vi "Teleop.vi"(10 "Match Info":T1={"Autonomous Elapsed Seconds"=0.0, "TeleOp Elapsed Seconds"=0.0, "Disabled Elapsed Seconds"=0.0, "Visited Autonomous"=FALSE, "Visited TeleOp"=FALSE, "Visited Disabled"=FALSE, "Autonomous Settings"={"Autonomous Style"=enum."Independent", "VI Refnum"=refnum}}, 11 "Call Context":T2) -> ()   [LabVIEW 2011]
doc: "This VI is called for each TeleOp packet received from the DS where the robot is not disabled. It is often used to read from the joysticks and update I/O or to update setpoints for timed control loops. It should complete and return within 20 milliseconds or it may miss DS packets."
uses:
  <vilib>/Rock Robotics/WPI/DriverStation/WPI_DriverStationDerivedRobotMode.ctl
  <vilib>/Rock Robotics/WPI/DriverStation/WPI_DriverStationMatch Info.ctl
  <vilib>/Rock Robotics/WPI/Relay/WPI_RelayValue.ctl
  <vilib>/Rock Robotics/WPI/DriverStation/DriverStationLCD/WPI_DriverStationLCDLCDLine.ctl
  Robot Global Data.vi
panel:
  in  "LDrive0":dbl
  in  "Rdrive0":dbl=0.9
  in  "Rdrive2":dbl=0.6
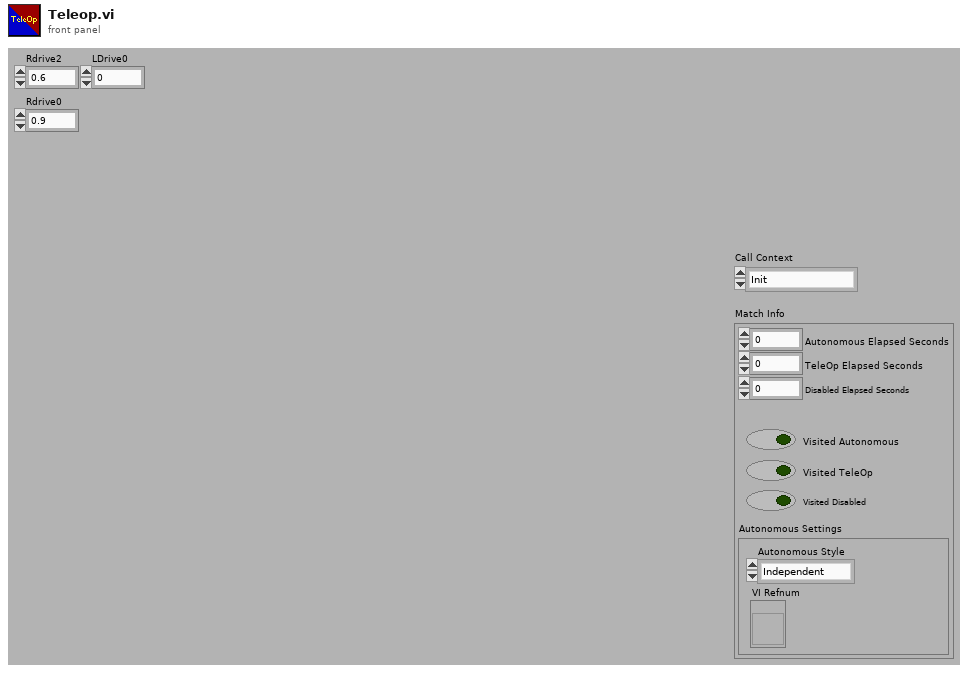
[diagram p1: front panel]
types:
  T1 = typedef "WPI_DriverStationMatch Info.ctl" = cluster{"Autonomous Elapsed Seconds":dbl, "TeleOp Elapsed Seconds":dbl, "Disabled Elapsed Seconds":dbl, "Visited Autonomous":bool, "Visited TeleOp":bool, "Visited Disabled":bool, "Autonomous Settings":cluster{"Autonomous Style":enum16{"Iterative", "Independent"}, "VI Refnum":refnum<vi>}}
  T2 = typedef "WPI_DriverStationDerivedRobotMode.ctl" = enum16{"Init", "Execute", "Stop"}
  T3 = typedef "WPI_RelayValue.ctl" = enum16{"Off", "On", "Forward", "Reverse"}
  T4 = typedef "WPI_JoystickDevRef.ctl" = cluster{"Device":T5}
  T5 = typedef "WPI_JoystickDeviceEnum.ctl" = enum16{"USB 1", "USB 2", "USB 3", "USB 4", "Kinect 1", "Kinect 2"}
  T6 = typedef "WPI_JoystickButtonState.ctl" = cluster{"Button 1":bool, "Button 2":bool, "Button 3":bool, "Button 4":bool, "Button 5":bool, "Button 6":bool, "Button 7":bool, "Button 8":bool, "Button 9":bool, "Button 10":bool, "Button 11":bool, "Button 12":bool}
  T7 = cluster{"axis 1 (x)":dbl, "axis 2 (y)":dbl, "axis 3 (throttle)":dbl, "axis 4":dbl, "axis 5":dbl, "axis 6":dbl}
  T8 = typedef "WPI_MotorControlDeviceRef.ctl" = cluster{"DeviceStatus":errorcluster, "Type":enum16{"PWM", "CAN"}, "PWM":cluster{"Digital Module":T9, "PWM Channel":T10, "DeadBand":T11}, "CAN":cluster{"Device Number":u8, "Control Mode":T12, "Semaphore":T13, "Max Vout":dbl}, "Invert":bool, "TransformRef":T14, "InvTransformRef":T14}
  T9 = typedef "FPGA_TypedefDigitalModule.ctl" = enum16{"Digital Module 1", "Digital Module 2"}
  T10 = typedef "FPGA_DIOPWMChannel.ctl" = enum8{"PWM 1", "PWM 2", "PWM 3", "PWM 4", "PWM 5", "PWM 6", "PWM 7", "PWM 8", "PWM 9", "PWM 10", "Invalid"}
  T11 = typedef "WPI_PWMDeadband.ctl" = cluster{"Name":string, "maxPositivePwm":i32, "minPositivePwm":i32, "centerPwm":i32, "maxNegativePwm":i32, "minNegativePwm":i32, "angularRange":u16}
  T12 = typedef "WPI_CANJaguar_ControlMode.ctl" = enum8{"Percent VBus", "Current", "Speed", "Position", "Voltage"}
  T13 = typedef "Semaphore RefNum" = refnum<k1>
  T14 = typedef "WPI_PWMTransform_ConPane.ctl" = refnum<vi>
  T15 = cluster{"Driver Station Digital Input (1-8)[0]":bool, "Driver Station Digital Input (1-8)[1]":bool, "Driver Station Digital Input (1-8)[2]":bool, "Driver Station Digital Input (1-8)[3]":bool, "Driver Station Digital Input (1-8)[4]":bool, "Driver Station Digital Input (1-8)[5]":bool, "Driver Station Digital Input (1-8)[6]":bool, "Driver Station Digital Input (1-8)[7]":bool, "Driver Station Digital Input (1-8)[8]":bool}
  T16 = typedef "WPI_RelayDevRef.ctl" = cluster{"DevStatus":errorcluster, "Relay Channel":T17, "Digital Module":T9, "Relay Direction":T18}
  T17 = typedef "FPGA_DIORelayChannel.ctl" = enum8{"Relay 1", "Relay 2", "Relay 3", "Relay 4", "Relay 5", "Relay 6", "Relay 7", "Relay 8", "Invalid"}
  T18 = typedef "WPI_RelayDirection.ctl" = enum16{"Both directions", "Forward only", "Reverse only"}
  T19 = typedef "WPI_DigitalInputDevRef.ctl" = cluster{"DevStatus":errorcluster, "DIO Channel":T20, "Digital Module":T9}
  T20 = typedef "FPGA_DIOChannel.ctl" = enum8{"DIO 1", "DIO 2", "DIO 3", "DIO 4", "DIO 5", "DIO 6", "DIO 7", "DIO 8", "DIO 9", "DIO 10", "DIO 11", "DIO 12", "DIO 13", "DIO 14", "Invalid"}
  T21 = typedef "WPI_EncoderDevRef.ctl" = cluster{"DevStatus":errorcluster, "EncoderIndex":T22, "CounterIndex":T23, "DistancePerCount":dbl, "Decoding Type":T24}
  T22 = typedef "FPGA_EncoderIdx.ctl" = enum8{"Enc 0", "Enc 1", "Enc 2", "Enc 3", "Invalid"}
  T23 = typedef "FPGA_CounterCtrSystemIndex.ctl" = enum8{"Ctr 0", "Ctr 1", "Ctr 2", "Ctr 3", "Ctr 4", "Ctr 5", "Ctr 6", "Ctr 7", "Invalid"}
  T24 = typedef "WPI_EncoderType.ctl" = enum16{"1x", "2x", "4x"}
  T25 = typedef "WPI_DriverStationLCDLCDLine.ctl" = enum16{"Main - Line 1", "User - Line 2", "User - Line 3", "User - Line 4", "User - Line 5", "User - Line 6"}
  T26 = typedef "WPI_ServoDeviceRef.ctl" = cluster{"DeviceStatus":errorcluster, "Digital Module":T9, "PWM Channel":T10, "DeadBand":T11}
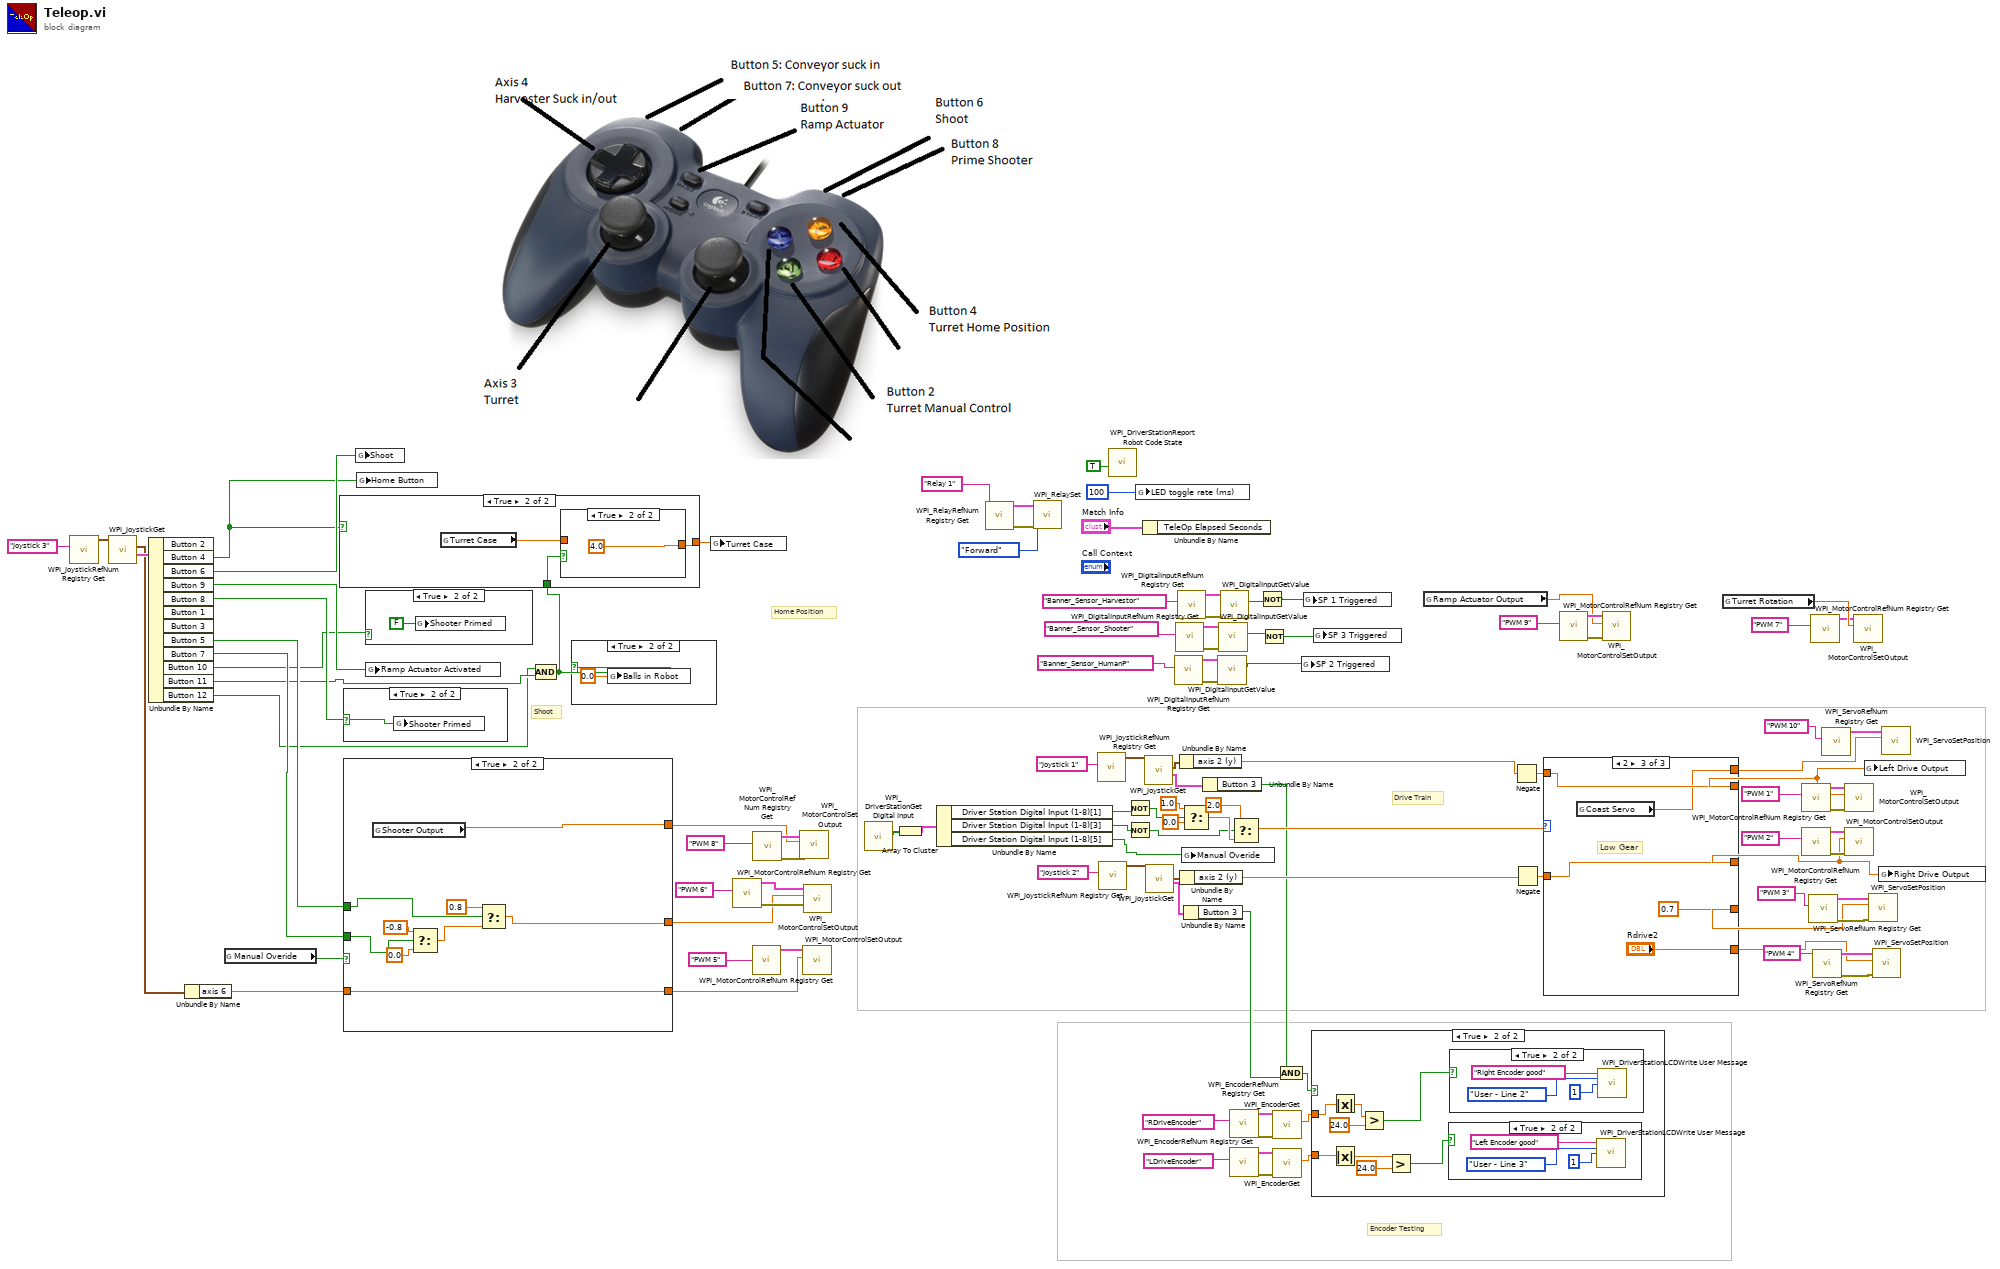
[diagram p0: block diagram]
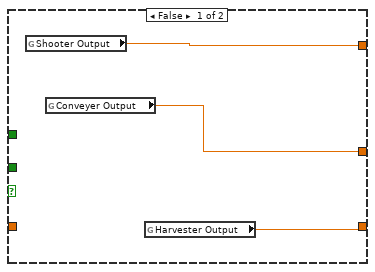
[diagram p7: hidden frame]
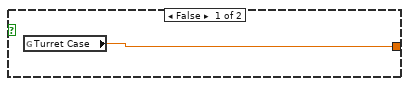
[diagram p9: hidden frame]
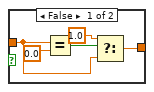
[diagram p10: hidden frame]
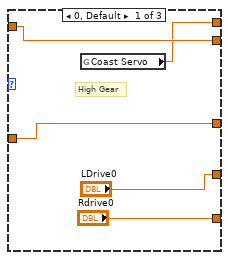
[diagram p11: hidden frame]
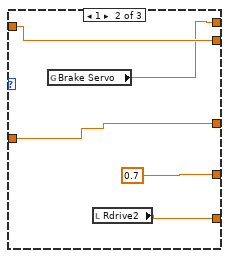
[diagram p12: hidden frame]
diagram:
  # "Encoder Testing"
  # "Shoot"
  # "Home Position"
  # "Drive Train"
  n1 = call <vilib>:"WPI_JoystickRefNum Registry Get.vi"("refnum name"="Joystick 3") -> ("JoystickDevRef"=w63:T4)  [unwired: 9 in, 1 out]
  n2 = call <vilib>:"WPI_JoystickGet.vi"("JoystickDevRef"=w63) -> ("Buttons"=w64:T6, "Axes"=w37:T7)  [unwired: 4 in, 1 out]
  n3 = Unbundle By Name(w64) -> ("Button 4"=w26:bool, "Button 6"=w62:bool, "Button 9"=w66:bool, "Button 8"=w38:bool, "Button 5"=w34:bool, "Button 7"=w33:bool, "Button 10"=w25:bool, "Button 11"=w24:bool, "Button 12"=w23:bool)  [unwired: 3 out]
  n4 = Unbundle By Name(w37) -> ("axis 6"=w21:dbl)
  n5 = global read "Robot Global Data.vi" "Manual Overide"() -> (w28:bool)
  n6 = case shown="True" w38 {
    selector: w38 -> [_ w111]
    frame False {
    }
    frame True {
      n7 = global write "Robot Global Data.vi" "Shooter Primed"(w111) -> ()
    }
  }
  n8 = case shown="True" w28 {
    tunnel: [w114 w115] -> w35
    tunnel: w34 -> [_ w118]
    tunnel: w33 -> [_ w119]
    tunnel: [w113 w117] -> w29
    tunnel: [w112 w116] -> w22
    tunnel: w21 -> [_ w116]
    frame False {
      n9 = global read "Robot Global Data.vi" "Shooter Output"() -> (w114:dbl)
      n10 = global read "Robot Global Data.vi" "Conveyer Output"() -> (w113:dbl)
      n11 = global read "Robot Global Data.vi" "Harvester Output"() -> (w112:dbl)
    }
    frame True {
      n12 = global read "Robot Global Data.vi" "Shooter Output"() -> (w115:dbl)
      n13 = Select(t=-0.8, s=w119, f=0.0) -> (s? t:f=w123:dbl)
      n14 = Select(t=0.8, s=w118, f=w123) -> (s? t:f=w117:dbl)
    }
  }
  n15 = global write "Robot Global Data.vi" "Shoot"(w62) -> ()
  n16 = global write "Robot Global Data.vi" "Home Button"(w26) -> ()
  n17 = case shown="True" w25 {
    frame False {
    }
    frame True {
      n18 = global write "Robot Global Data.vi" "Shooter Primed"(FALSE ("Shooter Primed")) -> ()
    }
  }
  n19 = global write "Robot Global Data.vi" "Ramp Actuator Activated"(w66) -> ()
  n20 = Compound Arithmetic op=AND(w23, w24) -> (w20:bool)
  n21 = case shown="True" w26 {
    tunnel: [w125 w126] -> w19
    tunnel: w20 -> [_ w128]
    frame False {
      n22 = global read "Robot Global Data.vi" "Turret Case"() -> (w125:dbl)
    }
    frame True {
      n23 = global read "Robot Global Data.vi" "Turret Case"() -> (w127:dbl)
      n24 = case shown="True" w128 {
        tunnel: w127 -> [w130 _]
        tunnel: [w129 4.0 ("Turret Case")] -> w126
        frame False {
          n25 = Equal?(x=w130, y=0.0) -> (x = y?=w132:bool)
          n26 = Select(t=1.0, s=w132, f=w130) -> (s? t:f=w129:dbl)
        }
        frame True {
        }
      }
    }
  }
  n27 = case shown="True" w20 {
    frame False {
    }
    frame True {
      n28 = global write "Robot Global Data.vi" "Balls in Robot"(0.0 ("Balls in Robot")) -> ()
    }
  }
  n29 = global write "Robot Global Data.vi" "Turret Case"(w19) -> ()
  n30 = call <vilib>:"WPI_MotorControlRefNum Registry Get.vi"("refnum name"="PWM 6") -> ("error out"=w30:errorcluster, "MotorControlDevRef"=w31:T8)  [unwired: 9 in]
  n31 = call <vilib>:"WPI_MotorControlRefNum Registry Get.vi"("refnum name"="PWM 5") -> ("MotorControlDevRef"=w56:T8)  [unwired: 9 in, 1 out]
  n32 = call <vilib>:"WPI_MotorControlRefNum Registry Get.vi"("refnum name"="PWM 8") -> ("error out"=w40:errorcluster, "MotorControlDevRef"=w41:T8)  [unwired: 9 in]
  n33 = call <vilib>:"WPI_MotorControlSetOutput.vi"("error in (no error)"=w40, "Output"=w35, "MotorControlDevRef"=w41) -> ()  [unwired: 7 in, 2 out]
  n34 = call <vilib>:"WPI_MotorControlSetOutput.vi"("Output"=w22, "MotorControlDevRef"=w56) -> ()  [unwired: 8 in, 2 out]
  n35 = call <vilib>:"WPI_MotorControlSetOutput.vi"("error in (no error)"=w30, "Output"=w29, "MotorControlDevRef"=w31) -> ()  [unwired: 7 in, 2 out]
  n36 = call <vilib>:"WPI_DriverStationGet Digital Input.vi"() -> ("Driver Station Digital Input (1-8)"=w85:bool[])  [unwired: 11 in]
  n37 = Array To Cluster(array=w85) -> (cluster=w107:T15)
  n38 = Unbundle By Name(w107) -> ("Driver Station Digital Input (1-8)[1]"=w88:bool, "Driver Station Digital Input (1-8)[3]"=w87:bool, "Driver Station Digital Input (1-8)[5]"=w1:bool)
  n39 = call <vilib>:"WPI_RelayRefNum Registry Get.vi"("refnum name"="Relay 1") -> ("error out"=w60:errorcluster, "RelayDevRef"=w61:T16)  [unwired: 9 in]
  n40 = call <vilib>:"WPI_RelaySet.vi"("error in (no error)"=w60, "RelayValue"=WPI_RelayValue."Forward", "RelayDevRef"=w61) -> ()  [unwired: 7 in, 2 out]
  n41 = call <vilib>:"WPI_JoystickRefNum Registry Get.vi"("refnum name"="Joystick 1") -> ("JoystickDevRef"=w100:T4)  [unwired: 9 in, 1 out]
  n42 = call <vilib>:"WPI_JoystickRefNum Registry Get.vi"("refnum name"="Joystick 2") -> ("JoystickDevRef"=w98:T4)  [unwired: 9 in, 1 out]
  n43 = call <vilib>:"WPI_DriverStationReport Robot Code State.vi"("TeleOp"=TRUE ("Autonomous")) -> ()  [unwired: 10 in, 1 out]
  n44 = Not(x=w88) -> (.not. x?=w86:bool)
  n45 = Not(x=w87) -> (.not. x?=w36:bool)
  n46 = global write "Robot Global Data.vi" "LED toggle rate (ms)"(u32 100 ("LED ms toggle rate")) -> ()
  n47 = Unbundle By Name("Match Info") -> ()  [unwired: 1 out]
  n48 = call <vilib>:"WPI_JoystickGet.vi"("JoystickDevRef"=w100) -> ("Buttons"=w16:T6, "Axes"=w17:T7)  [unwired: 4 in, 1 out]
  n49 = call <vilib>:"WPI_JoystickGet.vi"("JoystickDevRef"=w98) -> ("Buttons"=w18:T6, "Axes"=w99:T7)  [unwired: 4 in, 1 out]
  n50 = call <vilib>:"WPI_DigitalInputRefNum Registry Get.vi"("refnum name"="Banner_Sensor_HumanP") -> ("error out"=w51:errorcluster, "DigitalInputDevRef"=w50:T19)  [unwired: 9 in]
  n51 = call <vilib>:"WPI_DigitalInputRefNum Registry Get.vi"("refnum name"="Banner_Sensor_Shooter") -> ("error out"=w52:errorcluster, "DigitalInputDevRef"=w53:T19)  [unwired: 9 in]
  n52 = call <vilib>:"WPI_DigitalInputRefNum Registry Get.vi"("refnum name"="Banner_Sensor_Harvestor") -> ("error out"=w55:errorcluster, "DigitalInputDevRef"=w54:T19)  [unwired: 9 in]
  n53 = Unbundle By Name(w17) -> ("axis 2 (y)"=w84:dbl)
  n54 = Unbundle By Name(w99) -> ("axis 2 (y)"=w82:dbl)
  n55 = Select(t=1.0, s=w86, f=0.0 ("t")) -> (s? t:f=w104:dbl)
  n56 = global write "Robot Global Data.vi" "Manual Overide"(w1) -> ()
  n57 = Unbundle By Name(w18) -> ("Button 3"=w14:bool)
  n58 = Unbundle By Name(w16) -> ("Button 3"=w15:bool)
  n59 = call <vilib>:"WPI_DigitalInputGetValue.vi"("error in (no error)"=w51, "DigitalInputDevRef"=w50) -> ("Value"=w46:bool)  [unwired: 7 in, 2 out]
  n60 = call <vilib>:"WPI_DigitalInputGetValue.vi"("error in (no error)"=w52, "DigitalInputDevRef"=w53) -> ("Value"=w45:bool)  [unwired: 7 in, 2 out]
  n61 = call <vilib>:"WPI_DigitalInputGetValue.vi"("error in (no error)"=w55, "DigitalInputDevRef"=w54) -> ("Value"=w43:bool)  [unwired: 7 in, 2 out]
  n62 = call <vilib>:"WPI_EncoderRefNum Registry Get.vi"("refnum name"="RDriveEncoder") -> ("error out"=w10:errorcluster, "EncoderDevRef"=w11:T21)  [unwired: 9 in]
  n63 = call <vilib>:"WPI_EncoderRefNum Registry Get.vi"("refnum name"="LDriveEncoder") -> ("error out"=w9:errorcluster, "EncoderDevRef"=w8:T21)  [unwired: 9 in]
  n64 = Select(t=2.0, s=w36, f=w104) -> (s? t:f=w102:dbl)
  n65 = Not(x=w43) -> (.not. x?=w42:bool)
  n66 = Not(x=w45) -> (.not. x?=w44:bool)
  n67 = call <vilib>:"WPI_EncoderGet.vi"("error in (no error)"=w10, "EncoderDevRef"=w11) -> ("Distance"=w6:dbl)  [unwired: 4 in, 5 out]
  n68 = call <vilib>:"WPI_EncoderGet.vi"("error in (no error)"=w9, "EncoderDevRef"=w8) -> ("Distance"=w5:dbl)  [unwired: 4 in, 5 out]
  n69 = And(x=w15, y=w14) -> (x .and. y?=w13:bool)
  n70 = global write "Robot Global Data.vi" "SP 2 Triggered"(w46) -> ()
  n71 = global write "Robot Global Data.vi" "SP 1 Triggered"(w42) -> ()
  n72 = case shown="True" w13 {
    tunnel: w6 -> [_ w138]
    tunnel: w5 -> [_ w137]
    frame False {
    }
    frame True {
      n73 = Absolute Value(x=w138) -> (abs(x)=w139:dbl)
      n74 = Absolute Value(x=w137) -> (abs(x)=w136:dbl)
      n75 = Greater?(x=w139, y=24.0) -> (0:w142:bool)
      n76 = Greater?(x=w136, y=24.0) -> (0:w140:bool)
      n77 = case shown="True" w140 {
        frame False {
        }
        frame True {
          n78 = call <vilib>:"WPI_DriverStationLCDWrite User Message.vi"("line text"="Left Encoder good", "line"=WPI_DriverStationLCDLCDLine."User - Line 3", "starting column"=i8 1) -> ()  [unwired: 2 in, 11 out]
        }
      }
      n79 = case shown="True" w142 {
        frame False {
        }
        frame True {
          n80 = call <vilib>:"WPI_DriverStationLCDWrite User Message.vi"("line text"="Right Encoder good", "line"=WPI_DriverStationLCDLCDLine."User - Line 2", "starting column"=i8 1) -> ()  [unwired: 2 in, 11 out]
        }
      }
    }
  }
  n81 = global write "Robot Global Data.vi" "SP 3 Triggered"(w44) -> ()
  n82 = global read "Robot Global Data.vi" "Ramp Actuator Output"() -> (w27:dbl)
  n83 = Negate(x=w84) -> (-x=w83:dbl)
  n84 = Negate(x=w82) -> (-x=w81:dbl)
  n85 = case shown="2" w102 {
    tunnel: w81 -> [w154 w157 w164]
    tunnel: [w154 w157 w164] -> w73
    tunnel: [w153 w156 w163] -> w74
    tunnel: ["LDrive0" 0.7 0.7] -> w90
    tunnel: ["Rdrive0" w158 "Rdrive2"] -> w89
    tunnel: w83 -> [w153 w156 w163]
    tunnel: [w150 w155 w160] -> w2
    frame 0, Default {
      # "High Gear"
      n86 = global read "Robot Global Data.vi" "Coast Servo"() -> (w150:dbl)
    }
    frame 1 {
      n87 = global read "Robot Global Data.vi" "Brake Servo"() -> (w155:dbl)
      n88 = local read "Rdrive2"() -> (w158:dbl)
    }
    frame 2 {
      # "Low Gear"
      n89 = global read "Robot Global Data.vi" "Coast Servo"() -> (w160:dbl)
    }
  }
  n90 = call <vilib>:"WPI_MotorControlRefNum Registry Get.vi"("refnum name"="PWM 9") -> ("error out"=w71:errorcluster, "MotorControlDevRef"=w70:T8)  [unwired: 9 in]
  n91 = call <vilib>:"WPI_MotorControlSetOutput.vi"("error in (no error)"=w71, "Output"=w27, "MotorControlDevRef"=w70) -> ()  [unwired: 7 in, 2 out]
  n92 = global read "Robot Global Data.vi" "Turret Rotation"() -> (w69:dbl)
  n93 = call <vilib>:"WPI_MotorControlRefNum Registry Get.vi"("refnum name"="PWM 1") -> ("error out"=w78:errorcluster, "MotorControlDevRef"=w80:T8)  [unwired: 9 in]
  n94 = call <vilib>:"WPI_MotorControlRefNum Registry Get.vi"("refnum name"="PWM 2") -> ("error out"=w77:errorcluster, "MotorControlDevRef"=w76:T8)  [unwired: 9 in]
  n95 = call <vilib>:"WPI_ServoRefNum Registry Get.vi"("refnum name"="PWM 3") -> ("error out"=w94:errorcluster, "ServoDeviceRef"=w95:T26)  [unwired: 9 in]
  n96 = call <vilib>:"WPI_MotorControlRefNum Registry Get.vi"("refnum name"="PWM 7") -> ("MotorControlDevRef"=w67:T8)  [unwired: 9 in, 1 out]
  n97 = call <vilib>:"WPI_ServoRefNum Registry Get.vi"("refnum name"="PWM 4") -> ("error out"=w93:errorcluster, "ServoDeviceRef"=w92:T26)  [unwired: 9 in]
  n98 = call <vilib>:"WPI_ServoRefNum Registry Get.vi"("refnum name"="PWM 10") -> ("ServoDeviceRef"=w4:T26)  [unwired: 9 in, 1 out]
  n99 = call <vilib>:"WPI_MotorControlSetOutput.vi"("error in (no error)"=w78, "Output"=w74, "MotorControlDevRef"=w80) -> ()  [unwired: 7 in, 2 out]
  n100 = call <vilib>:"WPI_MotorControlSetOutput.vi"("error in (no error)"=w77, "Output"=w73, "MotorControlDevRef"=w76) -> ()  [unwired: 7 in, 2 out]
  n101 = call <vilib>:"WPI_MotorControlSetOutput.vi"("Output"=w69, "MotorControlDevRef"=w67) -> ()  [unwired: 8 in, 2 out]
  n102 = global write "Robot Global Data.vi" "Left Drive Output"(w74) -> ()
  n103 = call <vilib>:"WPI_ServoSetPosition.vi"("error in (no error)"=w94, "Position"=w90, "ServoDeviceRef"=w95) -> ()  [unwired: 7 in, 2 out]
  n104 = call <vilib>:"WPI_ServoSetPosition.vi"("error in (no error)"=w93, "Position"=w89, "ServoDeviceRef"=w92) -> ()  [unwired: 7 in, 2 out]
  n105 = global write "Robot Global Data.vi" "Right Drive Output"(w73) -> ()
  n106 = call <vilib>:"WPI_ServoSetPosition.vi"("Position"=w2, "ServoDeviceRef"=w4) -> ()  [unwired: 8 in, 2 out]
